vi "Average_Rotation_Tomography_v1.vi"(9 "Number of averages":u32, 11 "Summed data":T1) -> (0 "Data X/Y out":dbl[][](array[numeric]), 1 "Time":dbl[](array[numeric]), 2 "rotation spectrum":waveform(dbl)[](array[waveform]), 3 "rotation signal":cluster{"Time":dbl[], dbl[]}[](array[cluster]))   [LabVIEW 2021]
uses:
  Ver_1/Cutted_Data.ctl
  <vilib>/Analysis/NI_AALPro.lvlib
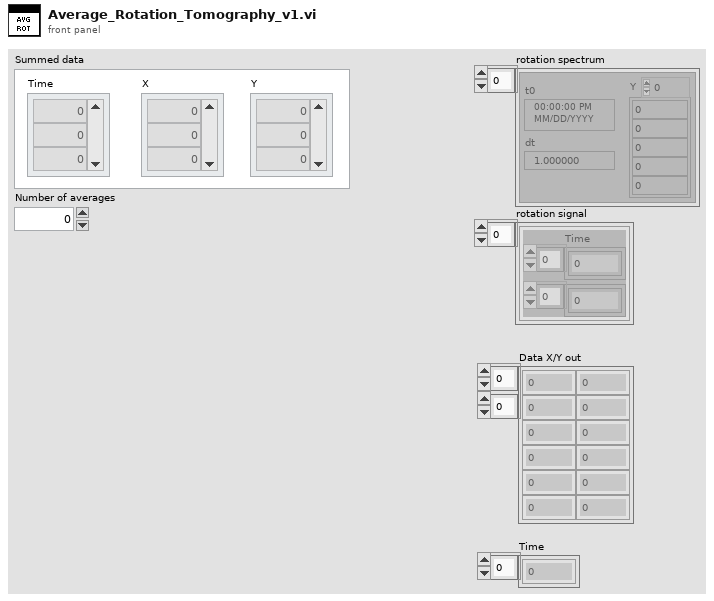
[diagram p1: front panel]
types:
  T1 = typedef "Cutted_Data.ctl" = cluster{"X":dbl[], "Y":dbl[], "Time":dbl[]}
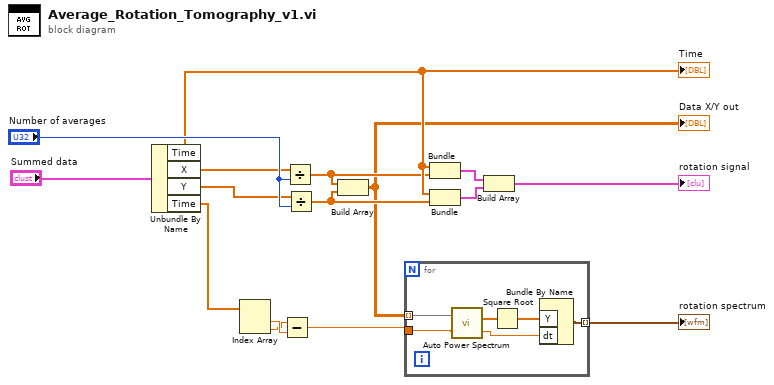
[diagram p0: block diagram]
diagram:
  n1 = Unbundle By Name("Summed data") -> ("Time"=w10:dbl[], "X"=w14:dbl[], "Y"=w13:dbl[], "Time"=w5:dbl[])
  "Time" <- w10
  n2 = Index Array(array=w5) -> (element #1=w2:dbl, element #2=w1:dbl)  [unwired: 2 in]
  n3 = Subtract(x=w1, y=w2) -> (x-y=w6:dbl)
  n4 = Divide(x=w14, y="Number of averages") -> (x/y=w9:dbl[])
  n5 = Divide(x=w13, y="Number of averages") -> (x/y=w7:dbl[])
  n6 = Build Array(w9, w7) -> (w4:dbl[][])
  "Data X/Y out" <- w4
  n7 = for {
    tunnel: w4 -> [w22] mode=indexing
    tunnel: w6 -> [w21]
    tunnel: [w17] -> w8 mode=indexing
    n8 = call <vilib>:"Auto Power Spectrum.vi"("dt"=w21, "Signal (V)"=w22) -> ("df"=w18:dbl, "Power Spectrum (V^2 rms)"=w20:dbl[])
    n9 = Square Root(x=w20) -> (sqrt(x)=w19:dbl[])
    n10 = Bundle By Name("Y"=w19, "dt"=w18) -> (w17:waveform(dbl))  [unwired: 1 in]
  }
  "rotation spectrum" <- w8
  n11 = Bundle("Time"=w10, w9) -> (w12:cluster{"Time":dbl[], dbl[]})  [unwired: 1 in]
  n12 = Bundle("Time"=w10, w7) -> (w11:cluster{"Time":dbl[], dbl[]})  [unwired: 1 in]
  n13 = Build Array(w12, w11) -> (→"rotation signal":cluster{"Time":dbl[], dbl[]}[])
